vi "Q_learning_Main.vi"() -> ()   [LabVIEW 2010]
uses:
  Q_learning_Global.vi
panel:
  out "Table Control":string[][](table)
  out "Title":string="LabVIEW and Q learning by all LabVIEW code"
  out "Q_table":dbl[][](array[numeric])
  out "step_counter":dbl=7.0
  out "episode":i32
  out "q_target":dbl
  out "q_predict":dbl
  out "Print":string="----OT"
  out "is_terminated":bool
  out "S (Position)":string="4"
  in  "Parameter":T1={"N_STATES"=7.0, "EPSILON"=0.9, "ALPHA"=0.1, "GAMMA"=0.9, "MAX_EPISODES"=18, "FRESH_TIME"=90.0, "ACTIONS"=["left", "right"]}
  # "left"
  # "right"
  # "1"
  # "2"
  # "3"
  # "4"
  # "5"
  # "6"
  # "7"
  # "8"
  # "Ricky"
  # "Reference : https://goo.gl/T6snvY"
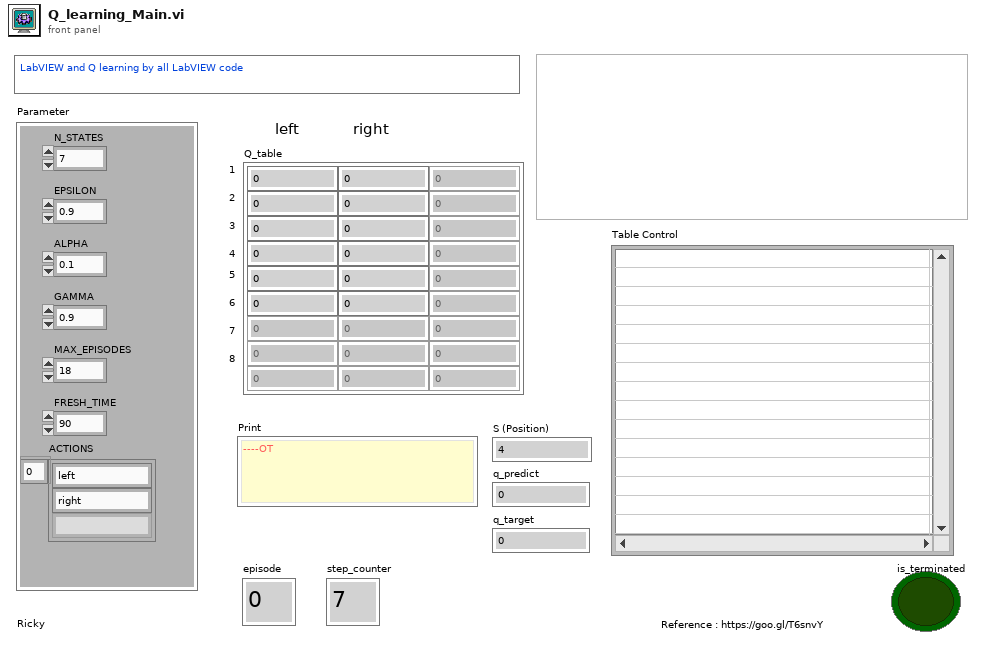
[diagram p1: front panel]
types:
  T1 = cluster{"N_STATES":dbl, "EPSILON":dbl, "ALPHA":dbl, "GAMMA":dbl, "MAX_EPISODES":i32, "FRESH_TIME":dbl, "ACTIONS":string[]}
  T2 = cluster{"N_STATES":dbl, "EPSILON":dbl, "ALPHA":dbl, "GAMMA":dbl, "MAX_EPISODES":dbl, "FRESH_TIME":dbl, "ACTIONS":string[]}
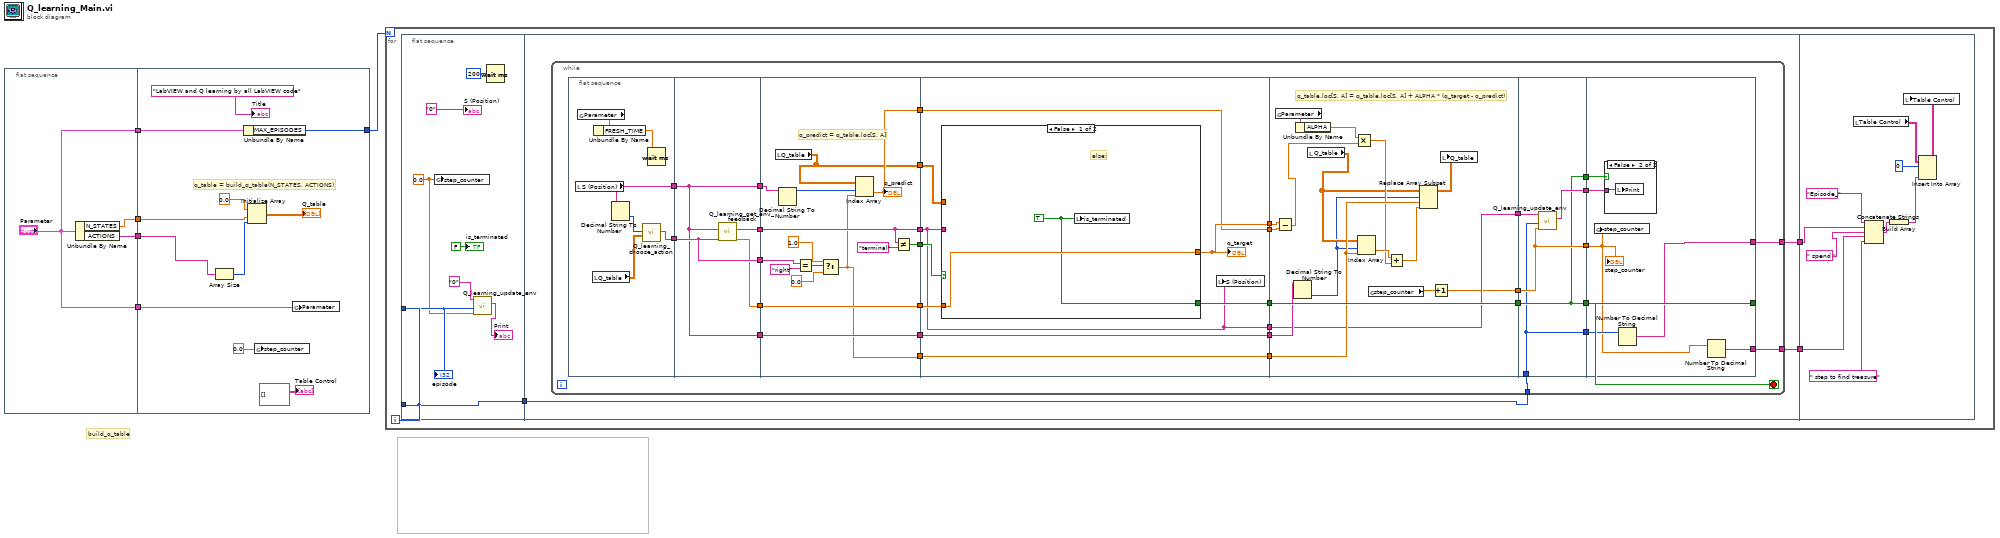
[diagram p0: block diagram]
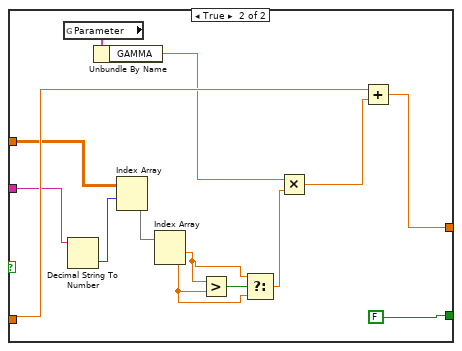
[diagram p2: hidden frame]
diagram:
  # "build_q_table"
  n1 = flat-sequence {
    tunnel: [w8] -> w5
    tunnel: [w7] -> w4
    tunnel: ["Parameter"] -> w3
    tunnel: ["Parameter"] -> w2
    tunnel: [w19] -> w1
    tunnel: w2 -> [w12]
    tunnel: w3 -> [w13]
    tunnel: w4 -> [w14]
    tunnel: w5 -> [w15]
    frame #0 {
      n2 = Unbundle By Name("Parameter") -> ("N_STATES"=w8:dbl, "ACTIONS"=w7:string[])
    }
    frame #1 {
      # "q_table = build_q_table(N_STATES, ACTIONS)"
      n3 = Array Size(array=w14) -> (size(s)=w17:i32)
      n4 = Unbundle By Name(w12) -> ("MAX_EPISODES"=w19:i32)
      n5 = Initialize Array(0.0 ("element"), w15, w17) -> (→"Q_table":dbl[][])
      n6 = global write "Q_learning_Global.vi" "step_counter"(0.0 ("step_counter")) -> ()
      n7 = global write "Q_learning_Global.vi" "Parameter"(w13) -> ()
      "Title" <- "LabVIEW and Q learning by all LabVIEW code" ("Title")
      "Table Control" <- string[][] [] ("Table Control")
    }
  }
  n8 = for {
    N: w1 -> [_]
    i -> [w22]
    n9 = flat-sequence {
      tunnel: w22 -> [w29]
      tunnel: [w25] -> w23
      tunnel: w22 -> [w25]
      tunnel: w23 -> [w34]
      tunnel: [w33] -> w21
      tunnel: [w32] -> w20
      tunnel: w21 -> [w150]
      tunnel: w20 -> [w148]
      frame #0 {
        w28 = 0.0 ("step_counter")
        n10 = global write "Q_learning_Global.vi" "step_counter"(w28) -> ()
        n11 = call "Q_learning_update_env.vi"("step_counter"=w28, "episode"=w29, "S"="0") -> ("Print"=→"Print":string)  [unwired: 8 in]
        n12 = Wait (ms)(milliseconds to wait=u32 200) -> ()  [unwired: 1 out]
        "is_terminated" <- FALSE ("is_terminated")
        "S (Position)" <- "0" ("S")
        "episode" <- w29
      }
      frame #1 {
        n13 = while {
          tunnel: w34 -> [w43]
          tunnel: [w36] -> w33
          tunnel: [w35] -> w32
          stop <- w56 stop-if-true
          n14 = flat-sequence {
            tunnel: [w71] -> w66
            tunnel: [w70] -> w65
            tunnel: w66 -> [w76]
            tunnel: w65 -> [w73]
            tunnel: [w73] -> w64
            tunnel: [w76] -> w63
            tunnel: [w75] -> w62
            tunnel: [w74] -> w59
            tunnel: [w73] -> w52
            tunnel: w64 -> [w91]
            tunnel: w63 -> [w88]
            tunnel: w62 -> [w81]
            tunnel: [w83] -> w61
            tunnel: [w82] -> w60
            tunnel: w59 -> [w82]
            tunnel: [w77] -> w58
            tunnel: [w81] -> w57
            tunnel: [w80] -> w53
            tunnel: w52 -> [w80]
            tunnel: [w79] -> w50
            tunnel: [w78] -> w46
            tunnel: w61 -> [w100]
            tunnel: w60 -> [w99]
            tunnel: w58 -> [w98]
            tunnel: w57 -> [w92]
            tunnel: [w97] -> w55
            tunnel: [w96] -> w54
            tunnel: w53 -> [w96]
            tunnel: [w95] -> w51
            tunnel: w50 -> [w95]
            tunnel: [w94] -> w48
            tunnel: [w93] -> w47
            tunnel: w46 -> [w93]
            tunnel: [w92] -> w44
            tunnel: w55 -> [w133]
            tunnel: w54 -> [w132]
            tunnel: w51 -> [w130]
            tunnel: [w133] -> w49
            tunnel: w48 -> [w126]
            tunnel: w47 -> [w125]
            tunnel: [w122] -> w45
            tunnel: w44 -> [w122]
            tunnel: [w120] -> w42
            tunnel: w49 -> [w135]
            tunnel: w45 -> [w138]
            tunnel: w43 -> [w134]
            tunnel: w42 -> [w137]
            tunnel: [w135] -> w41
            tunnel: [w137] -> w40
            tunnel: [w136] -> w39
            tunnel: [w135] -> w38
            tunnel: [w134] -> w37
            tunnel: [w145] -> w56
            tunnel: w41 -> [w145]
            tunnel: w40 -> [w140]
            tunnel: w39 -> [w144]
            tunnel: w38 -> [w143]
            tunnel: w37 -> [w142]
            tunnel: [w141] -> w36
            tunnel: [w139] -> w35
            frame #0 {
              n15 = local read "S (Position)"() -> (w70:string)
              n16 = global read "Q_learning_Global.vi" "Parameter"() -> (w68:T2)
              n17 = local read "Q_table"() -> (w69:dbl[][])
              n18 = Unbundle By Name(w68) -> ("FRESH_TIME"=w67:dbl)
              n19 = Decimal String To Number(string=w70) -> (number=w72:i32)  [unwired: 2 in, 1 out]
              n20 = call "Q_learning_choose_action.vi"("Q_table"=w69, "state"=w72) -> ("action_name"=w71:string)  [unwired: 9 in]
              n21 = Wait (ms)(milliseconds to wait=w67) -> ()  [unwired: 1 out]
            }
            frame #1 {
              n22 = call "Q_learning_get_env_feedback.vi"("A"=w76, "S"=w73) -> ("R"=w74:dbl, "S_"=w75:string)  [unwired: 8 in]
            }
            frame #2 {
              # "q_predict = q_table.loc[S, A]"
              n23 = local read "Q_table"() -> (w77:dbl[][])
              n24 = Decimal String To Number(string=w91) -> (number=w90:i32)  [unwired: 2 in, 1 out]
              n25 = Equal?(x=w88, y="right") -> (x = y?=w87:bool)
              n26 = Select(t=1.0, s=w87, f=0.0 ("t")) -> (s? t:f=w79:dbl)
              n27 = Index Array(array=w77, index (row)=w90, index (col)=w79) -> (element=w78:dbl)
              "q_predict" <- w78
              n28 = Not Equal?(x=w81, y="terminal") -> (x != y?=w83:bool)
            }
            frame #3 {
              n29 = case shown="False" w100 {
                tunnel: w99 -> [w102 w116]
                tunnel: [w102 w104] -> w94
                tunnel: w98 -> [_ w113]
                tunnel: w92 -> [_ w112]
                tunnel: [w101 FALSE ("is_terminated")] -> w97
                frame False {
                  w101 = TRUE ("is_terminated")
                  # "else:"
                  n30 = local write "is_terminated"(w101) -> ()
                }
                frame True {
                  n31 = global read "Q_learning_Global.vi" "Parameter"() -> (w115:T2)
                  n32 = Decimal String To Number(string=w112) -> (number=w111:i32)  [unwired: 2 in, 1 out]
                  n33 = Unbundle By Name(w115) -> ("GAMMA"=w114:dbl)
                  n34 = Index Array(array=w113, index (row)=w111) -> (element=w110:dbl[])  [unwired: 1 in]
                  n35 = Index Array(array=w110) -> (element #1=w108:dbl, element #2=w107:dbl)  [unwired: 2 in]
                  n36 = Greater?(x=w108, y=w107) -> (0:w109:bool)
                  n37 = Select(t=w108, s=w109, f=w107) -> (s? t:f=w106:dbl)
                  n38 = Multiply(x=w114, y=w106) -> (x*y=w105:dbl)
                  n39 = Add(x=w116, y=w105) -> (x+y=w104:dbl)
                }
              }
              "q_target" <- w94
              n40 = local write "S (Position)"(w92) -> ()
            }
            frame #4 {
              # "q_table.loc[S, A] = q_table.loc[S, A] + ALPHA * (q_target - q_predict)"
              n41 = global read "Q_learning_Global.vi" "Parameter"() -> (w128:T2)
              n42 = Subtract(x=w126, y=w125) -> (x-y=w124:dbl)
              n43 = Decimal String To Number(string=w132) -> (number=w117:i32)  [unwired: 2 in, 1 out]
              n44 = Unbundle By Name(w128) -> ("ALPHA"=w127:dbl)
              n45 = local read "Q_table"() -> (w119:dbl[][])
              n46 = Multiply(x=w127, y=w124) -> (x*y=w123:dbl)
              n47 = Index Array(array=w119, index (row)=w117, index (col)=w130) -> (element=w131:dbl)
              n48 = global read "Q_learning_Global.vi" "step_counter"() -> (w121:dbl)
              n49 = Add(x=w131, y=w123) -> (x+y=w129:dbl)
              n50 = Replace Array Subset "Replace Array Subset"(array=w119, new element=w129, index (row)=w117, index (col)=w130) -> (w118:dbl[][])
              n51 = Increment(x=w121) -> (x+1=w120:dbl)
              n52 = local write "Q_table"(w118) -> ()
            }
            frame #5 {
              n53 = call "Q_learning_update_env.vi"("step_counter"=w137, "episode"=w134, "S"=w138) -> ("Print"=w136:string)  [unwired: 8 in]
            }
            frame #6 {
              n54 = global write "Q_learning_Global.vi" "step_counter"(w140) -> ()
              n55 = case shown="False" w143 {
                tunnel: w144 -> [_ w146]
                frame True {
                }
                frame False {
                  n56 = local write "Print"(w146) -> ()
                }
              }
              n57 = Number To Decimal String(number=w142) -> (decimal integer string=w141:string)  [unwired: 1 in]
              n58 = Number To Decimal String(number=w140) -> (decimal integer string=w139:string)  [unwired: 1 in]
              "step_counter" <- w140
            }
          }
        }
      }
      frame #2 {
        n59 = local read "Table Control"() -> (w156:string[][])
        n60 = Concatenate Strings("Episode_" ("string"), w150, " spend " ("string"), w148, " step to find treasure" ("string")) -> (w153:string)
        n61 = Build Array(w153) -> (w152:string[])
        n62 = Insert Into Array(array=w156, index (row)=0, new element=w152) -> (w155:string[][])  [unwired: 1 in]
        n63 = local write "Table Control"(w155) -> ()
      }
    }
  }
